vi "Two Button Dialog with Icon.vi"(6 "Toggle Key Shortcut (<Return>,<Esc>":T1(array[cluster])=[{"Focus"=FALSE, "Control"=FALSE, "Shift"=FALSE, "Key"="<Return>"}, {"Focus"=FALSE, "Control"=FALSE, "Shift"=FALSE, "Key"="<Escape>"}], 7 "Window Title (\"\")":string, 8 "Symbol":T2=enum."Warning", 9 "F button name (\"Cancel\")":string="Cancel", 10 "T button name (\"OK\")":string="OK", 11 "Message":string) -> (3 "T Button?":bool)   [LabVIEW 2014, in "Modbus System Explorer.lvlib"]
uses:
  Modbus System Explorer.lvlib
  Shared/3_But_Dlg_Symbol.ctl
  Shared/3_But_Which_Button.ctl
  Shared/Modbus Shared.lvlib
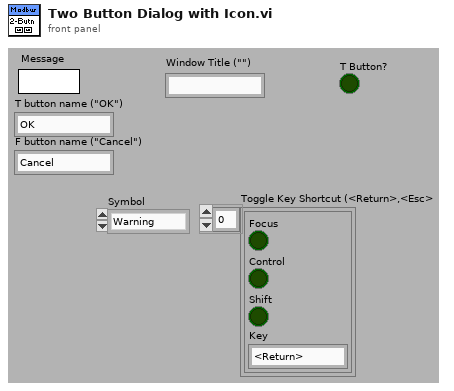
[diagram p1: front panel]
types:
  T1 = cluster{"Focus":bool, "Control":bool, "Shift":bool, "Key":string}[]
  T2 = typedef "Modbus Shared.lvlib/3_But_Dlg_Symbol.ctl" = enum16{"Information", "Help", "Warning", "Error"}
  T3 = typedef "Modbus Shared.lvlib/3_But_Which_Button.ctl" = enum16{"Left Button", "Center Button", "Right Button", "Window Close"}
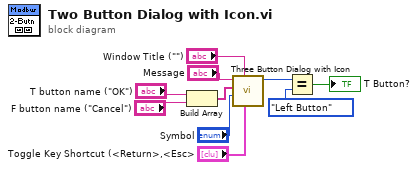
[diagram p0: block diagram]
diagram:
  n1 = Build Array("T button name (\"OK\")", "F button name (\"Cancel\")") -> (w1:string[])
  n2 = call "Three Button Dialog with Icon.vi"("Toggle Key Shortcut (<Return>, , <Esc>"="Toggle Key Shortcut (<Return>,<Esc>", "Window Title (\"\")"="Window Title (\"\")", "Symbol"="Symbol", "Button Strings"=w1, "Message"="Message") -> ("Which Button?"=w6:T3)  [unwired: 2 in, 4 out]
  n3 = Equal?(x=w6, y=3_But_Which_Button."Left Button") -> (x = y?=→"T Button?":bool)
